vi "encode output.vi"(10 "data":T1, 11 "DGUS输入":refnum<class "DGUS.lvclass">) -> (2 "数据帧":string, 3 "DGUS输出":refnum<class "DGUS.lvclass">)   [LabVIEW 2016, in "DGUS.lvlib" / "DGUS.lvclass"]
uses:
  DGUS.lvclass
  DGUS.lvclass/DGUS.ctl
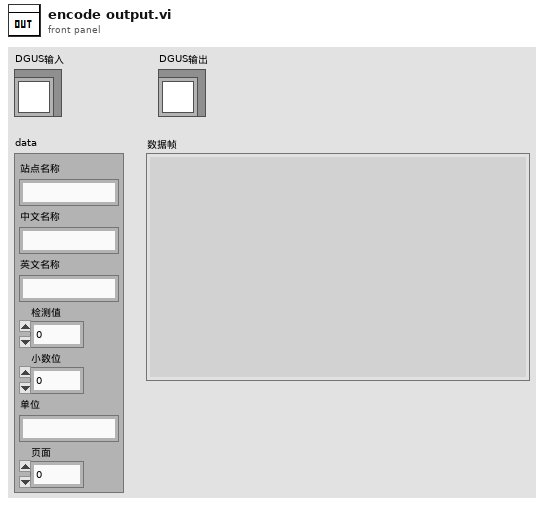
[diagram p1: front panel]
types:
  T1 = cluster{"站点名称":string, "中文名称":string, "英文名称":string, "检测值":sgl, "小数位":u8, "单位":string, "页面":u16}
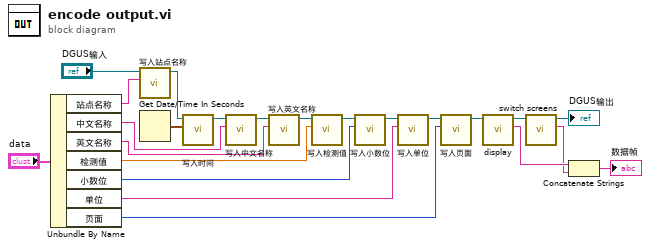
[diagram p0: block diagram]
diagram:
  n1 = Unbundle By Name("data") -> ("站点名称"=w10:string, "中文名称"=w9:string, "英文名称"=w8:string, "检测值"=w7:sgl, "小数位"=w6:u8, "单位"=w5:string, "页面"=w4:u16)
  n2 = call "写入站点名称.vi"("站点名称"=w10, "DGUS输入"="DGUS输入") -> ("DGUS输出"=w19:refnum<class "DGUS.lvclass">)  [unwired: 8 in, 1 out]
  n3 = Get Date/Time In Seconds() -> (seconds since 1Jan1904=w22:timestamp)
  n4 = call "写入时间.vi"("时间"=w22, "DGUS输入"=w19) -> ("DGUS输出"=w18:refnum<class "DGUS.lvclass">)  [unwired: 8 in, 1 out]
  n5 = call "写入中文名称.vi"("中文名称"=w9, "DGUS输入"=w18) -> ("DGUS输出"=w17:refnum<class "DGUS.lvclass">)  [unwired: 8 in, 1 out]
  n6 = call "写入英文名称.vi"("英文名称"=w8, "DGUS输入"=w17) -> ("DGUS输出"=w16:refnum<class "DGUS.lvclass">)  [unwired: 8 in, 1 out]
  n7 = call "写入检测值.vi"("检测值"=w7, "DGUS输入"=w16) -> ("DGUS输出"=w15:refnum<class "DGUS.lvclass">)  [unwired: 8 in, 1 out]
  n8 = call "写入小数位.vi"("小数位"=w6, "DGUS输入"=w15) -> ("DGUS输出"=w14:refnum<class "DGUS.lvclass">)  [unwired: 8 in, 1 out]
  n9 = call "写入单位.vi"("单位"=w5, "DGUS输入"=w14) -> ("DGUS输出"=w13:refnum<class "DGUS.lvclass">)  [unwired: 8 in, 1 out]
  n10 = call "写入页面.vi"("页面"=w4, "DGUS输入"=w13) -> ("DGUS输出"=w12:refnum<class "DGUS.lvclass">)  [unwired: 8 in, 1 out]
  n11 = call "display.vi"("DGUS 输入"=w12) -> ("字符串"=w3:string, "DGUS 输出"=w21:refnum<class "DGUS.lvclass">)  [unwired: 8 in, 1 out]
  n12 = call "switch screens.vi"("DGUS 输入"=w21) -> ("字符串"=w2:string, "DGUS 输出"=→"DGUS输出":refnum<class "DGUS.lvclass">)  [unwired: 8 in, 1 out]
  n13 = Concatenate Strings(w3, w2) -> (→"数据帧":string)
